vi "addcomma.vi"(10 "INPUT":string) -> (2 "OUTPUT":string)   [LabVIEW 2012]
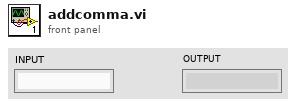
[diagram p1: front panel]
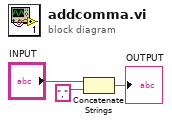
[diagram p0: block diagram]
diagram:
  n1 = Concatenate Strings("INPUT", ",") -> (→"OUTPUT":string)
